vi "RTS Macro Extract Compressor Cycles.vi"(0 "Full Time":dbl[](array[numeric]), 5 "Full Power Factor Data":dbl[](array[numeric]), 7 "Full Power Data":dbl[](array[numeric]), 9 "Full WH Data":dbl[](array[numeric]), 11 "Error In":errorcluster) -> (4 "Filtered Time":dbl[](array[numeric]), 6 "Filtered Power Factor":dbl[](array[numeric]), 8 "Filtered Power Data":dbl[](array[numeric]), 10 "Filtered Wh Data":dbl[](array[numeric]), 13 "Filtered Pulse Train":dbl[](array[numeric]), 14 "Top Compressor Range Data":dbl, 15 "Error Out":errorcluster)   [LabVIEW 2016]
uses:
  <vilib>/Analysis/NI_AALBase.lvlib
panel:
  out "Histogram Graph":T1(graph)
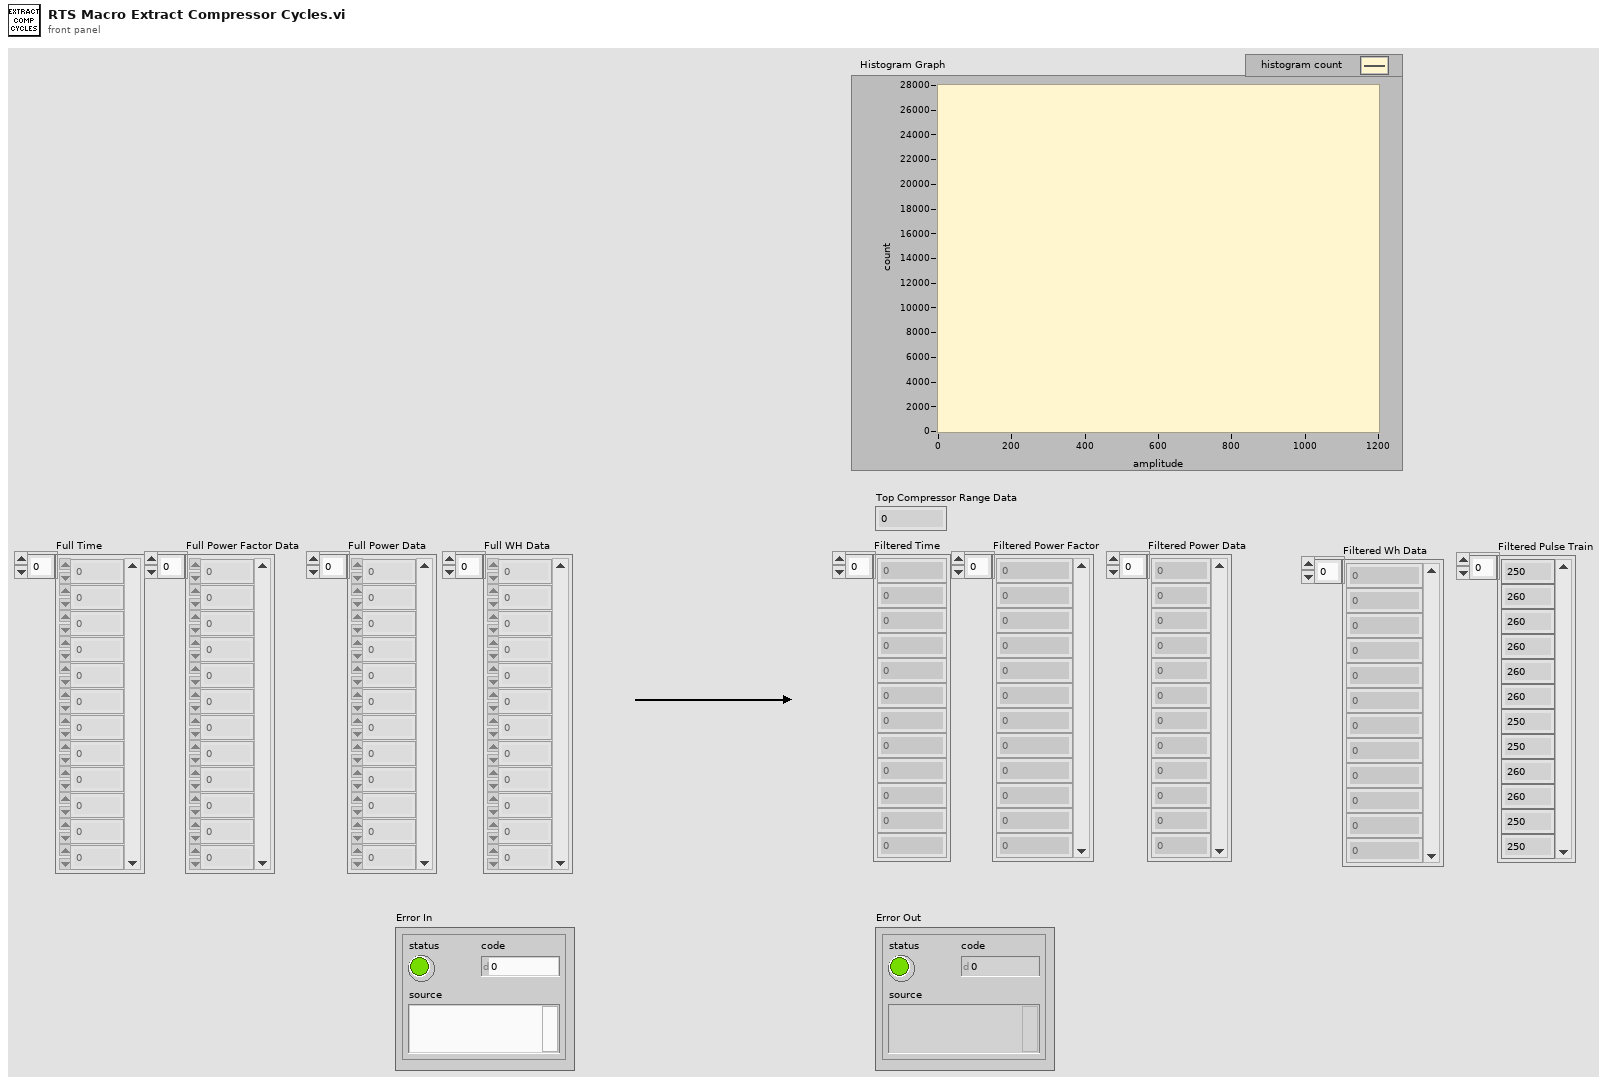
[diagram p1: front panel]
types:
  T1 = cluster{"X Values":dbl[], "Histogram: h(x)":i32[]}
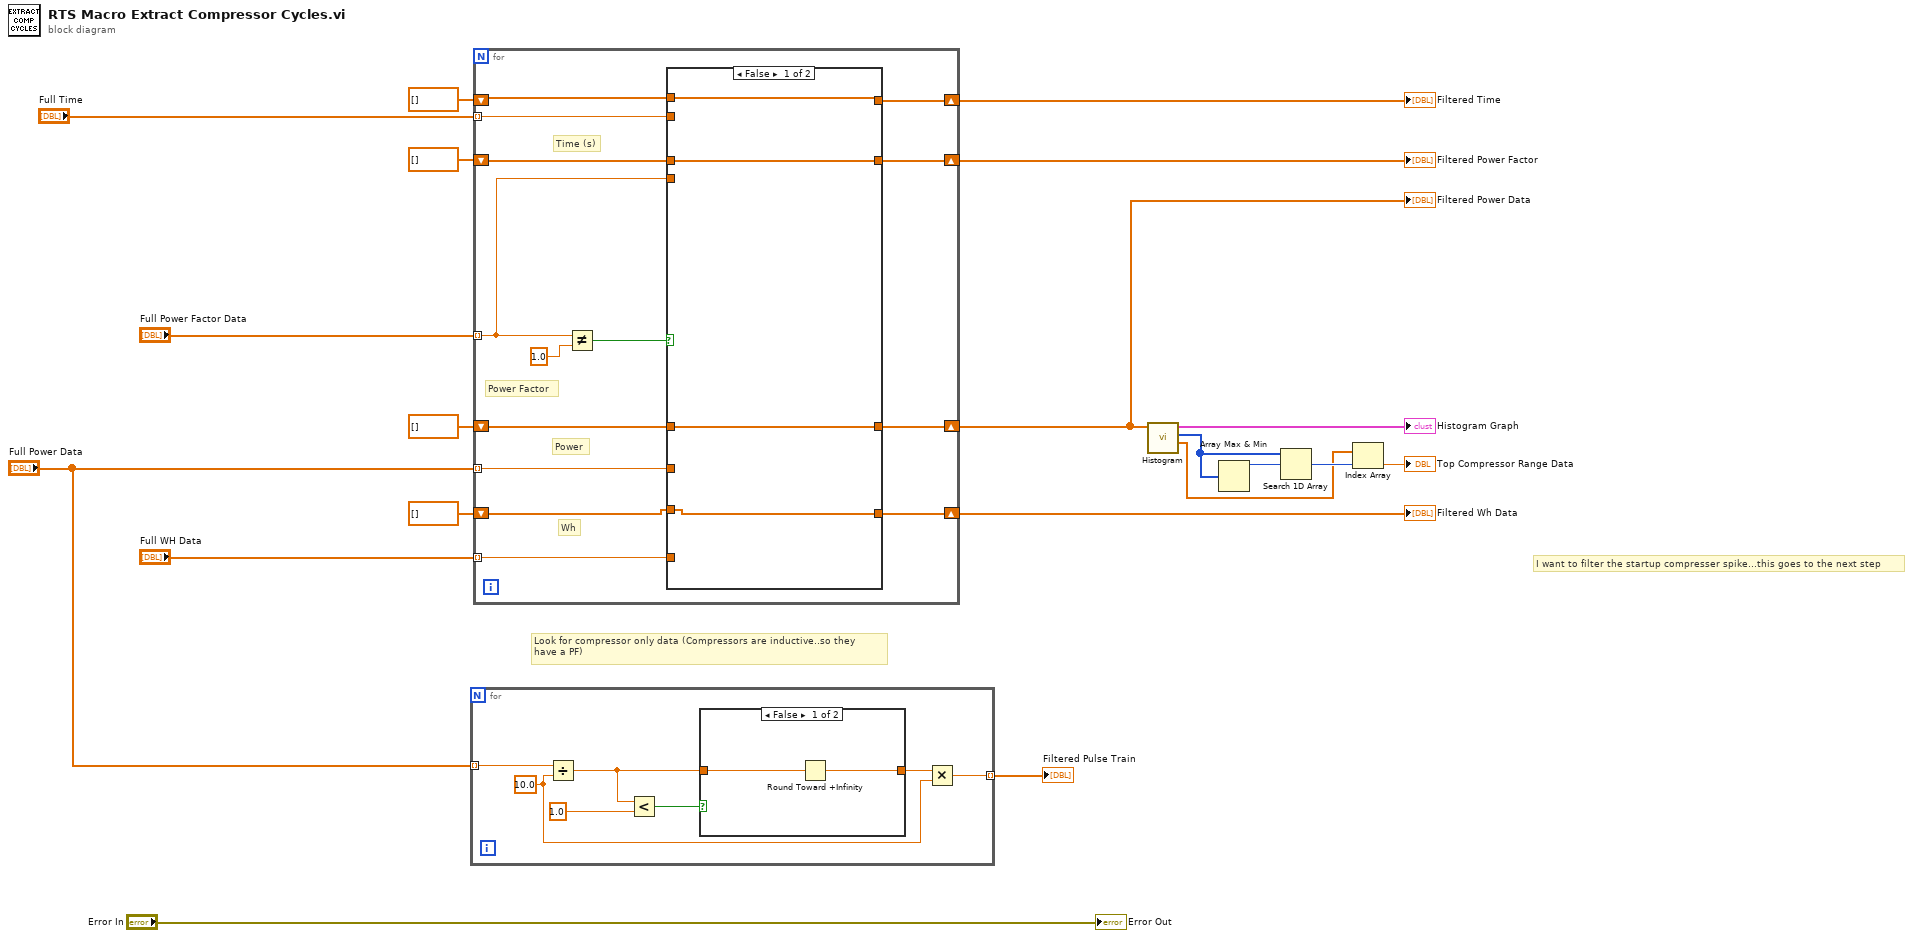
[diagram p0: block diagram]
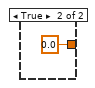
[diagram p2: hidden frame]
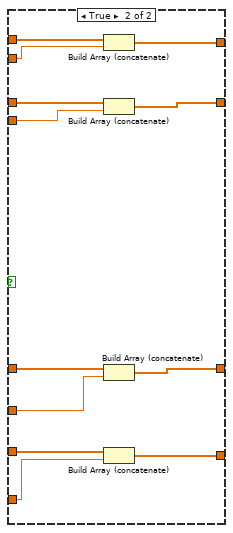
[diagram p3: hidden frame]
diagram:
  # "I want to filter the startup compresser spike...this goes to the next step"
  # "Look for compressor only data (Compressors are inductive..so they\nhave a PF)"
  n1 = for {
    tunnel: "Full Power Data" -> [w27] mode=indexing
    tunnel: [w22] -> w1 mode=indexing
    w21 = 10.0 ("y")
    n2 = Divide(x=w27, y=w21) -> (x/y=w24:dbl)
    n3 = Less?(x=w24, y=1.0) -> (x < y?=w25:bool)
    n4 = case shown="False" w25 {
      tunnel: w24 -> [w29 _]
      tunnel: [w28 0.0] -> w23
      frame False {
        n5 = Round Toward +Infinity(x=w29) -> (ceil(x): smallest int >= x=w28:dbl)
      }
      frame True {
      }
    }
    n6 = Multiply(x=w23, y=w21) -> (x*y=w22:dbl)
  }
  "Filtered Pulse Train" <- w1
  n7 = for {
    tunnel: "Full Power Factor Data" -> [w33] mode=indexing
    shift-right: [w43] -> w20
    shift-left: dbl[] [] -> [w44]
    shift-right: [w41] -> w15
    shift-left: dbl[] [] -> [w42]
    tunnel: "Full Power Data" -> [w40] mode=indexing
    shift-right: [w38] -> w19
    shift-left: dbl[] [] -> [w39]
    tunnel: "Full WH Data" -> [w37] mode=indexing
    tunnel: "Full Time" -> [w34] mode=indexing
    shift-right: [w35] -> w17
    shift-left: dbl[] [] -> [w36]
    # "Wh"
    # "Power"
    # "Power Factor"
    # "Time (s)"
    n8 = Not Equal?(x=w33, y=1.0) -> (x != y?=w31:bool)
    n9 = case shown="False" w31 {
      tunnel: w44 -> [w48 w60]
      tunnel: [w48 w59] -> w43
      tunnel: w33 -> [_ w58]
      tunnel: w42 -> [w47 w57]
      tunnel: [w47 w56] -> w41
      tunnel: w40 -> [_ w49]
      tunnel: w39 -> [w46 w55]
      tunnel: [w46 w54] -> w38
      tunnel: w37 -> [_ w53]
      tunnel: w36 -> [w45 w52]
      tunnel: [w45 w51] -> w35
      tunnel: w34 -> [_ w50]
      frame False {
      }
      frame True {
        n10 = Build Array (concatenate)(w52, w50) -> (w51:dbl[])
        n11 = Build Array (concatenate)(w60, w58) -> (w59:dbl[])
        n12 = Build Array (concatenate)(w57, w49) -> (w56:dbl[])
        n13 = Build Array (concatenate)(w55, w53) -> (w54:dbl[])
      }
    }
  }
  "Filtered Power Factor" <- w20
  "Filtered Wh Data" <- w19
  "Filtered Time" <- w17
  "Filtered Power Data" <- w15
  n14 = call <vilib>:"Histogram.vi"("X"=w15) -> ("X Values"=w13:dbl[], "Histogram: h(x)"=w11:i32[], "Histogram Graph"=→"Histogram Graph":T1)  [unwired: 7 in, 1 out]
  n15 = Array Max & Min(array=w11) -> (max value=w12:i32)  [unwired: 3 out]
  n16 = Search 1D Array(1D array=w11, element=w12) -> (index of element=w14:i32)  [unwired: 1 in]
  n17 = Index Array(array=w13, index=w14) -> (element=→"Top Compressor Range Data":dbl)
  "Error Out" <- "Error In"
